vi "ImageAnalysis.vi"(8 "error in (no error)":errorcluster, 10 "config":T5, 11 "data":T1) -> (0 "error out":errorcluster, 3 "data out":T1)   [LabVIEW 2017, in "IrAnalysis.lvlib"]
uses:
  <vilib>/addons/InsightCM/Devices/Shared/Ir/IrAnalysis/IrAnalysis.lvlib
  <vilib>/addons/InsightCM/Devices/Shared/Common/DataFlow/controls/Data.ctl
  <vilib>/addons/InsightCM/Utilities/DataAccessors/controls/wfmSGL_DVR.ctl
  <vilib>/addons/PointValueMap/controls/PointMap.ctl
  <vilib>/addons/InsightCM/Devices/Shared/Common/DataFlow/controls/Type.ctl
  <vilib>/addons/InsightCM/Devices/Shared/Ir/IrAnalysis/controls/config.ctl
  <vilib>/addons/InsightCM/Devices/Shared/Ir/IrAnalysis/controls/roi.ctl
  <vilib>/addons/InsightCM/Devices/Shared/Ir/IrAnalysis/controls/metric.ctl
  <vilib>/addons/InsightCM/MessageBus/Base/controls/MetricDefinitionInstance.ctl
  <vilib>/addons/InsightCM/MessageBus/Base/controls/KeyValuePair.ctl
  <vilib>/addons/PointValueMap/PointValueMap.lvlib
  <vilib>/addons/InsightCM/Devices/Shared/Common/DataFlow/DataFlow.lvlib
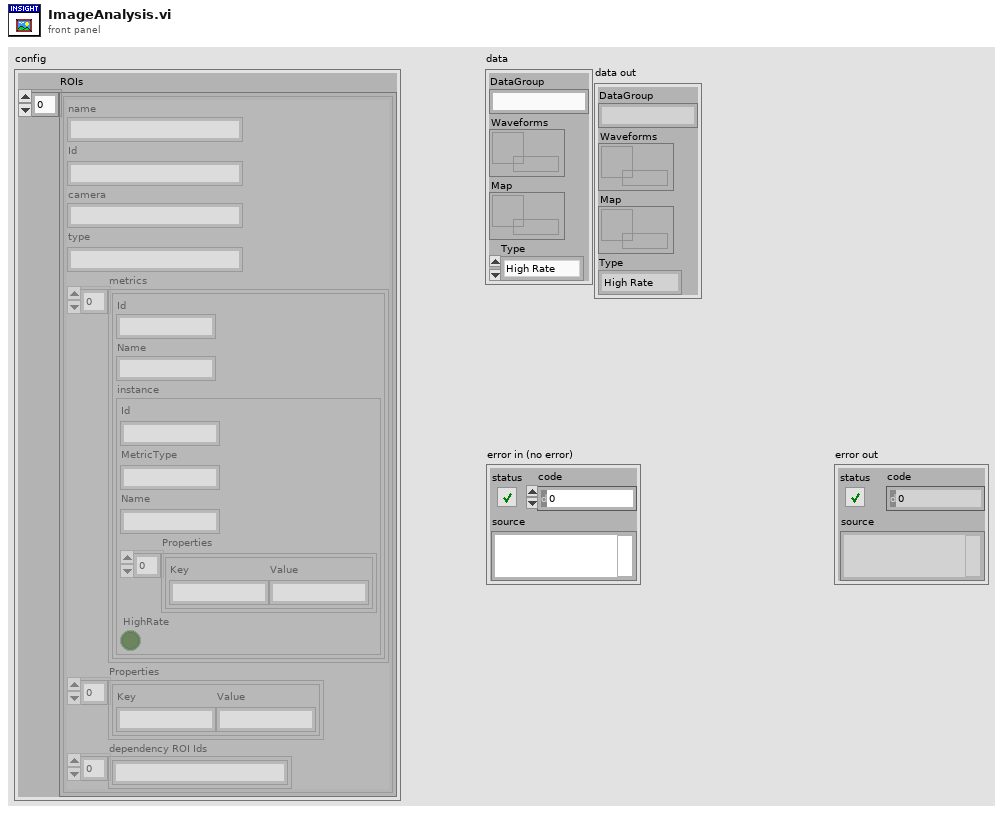
[diagram p1: front panel]
types:
  T1 = typedef "DataFlow.lvlib/Data.ctl" = cluster{"DataGroup":string, "Waveforms":T2, "Map":T3, "Type":T4}
  T2 = typedef "wfmSGL_DVR.ctl" = refnum<data-value>
  T3 = typedef "PointValueMap.lvlib/PointMap.ctl" = refnum<data-value>
  T4 = typedef "DataFlow.lvlib/Type.ctl" = enum16{"High Rate", "Low Rate", "Burst Mode"}
  T5 = typedef "IrAnalysis.lvlib/config.ctl" = cluster{"ROIs":T6[]}
  T6 = typedef "IrAnalysis.lvlib/roi.ctl" = cluster{"name":string, "Id":string, "camera":string, "type":string, "metrics":T7[], "Properties":T9[], "dependency ROI Ids":string[]}
  T7 = typedef "IrAnalysis.lvlib/metric.ctl" = cluster{"Id":string, "Name":string, "instance":T8}
  T8 = typedef "MetricDefinitionInstance.ctl" = cluster{"Id":string, "MetricType":string, "Name":string, "Properties":T9[], "HighRate":bool}
  T9 = typedef "KeyValuePair.ctl" = cluster{"Key":string, "Value":string}
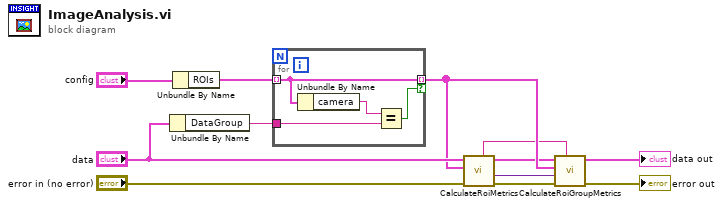
[diagram p0: block diagram]
diagram:
  n1 = Unbundle By Name("data") -> ("DataGroup"=w12:string)
  n2 = Unbundle By Name("config") -> ("ROIs"=w9:T6[])
  n3 = for {
    tunnel: w9 -> [w14] mode=indexing
    tunnel: w12 -> [w15]
    tunnel: [w14] -> w4 mode=indexing if=w13
    n4 = Unbundle By Name(w14) -> ("camera"=w16:string)
    n5 = Equal?(x=w16, y=w15) -> (x = y?=w13:bool)
  }
  n6 = call <vilib>:"CalculateRoiMetrics.vi"("error in (no error)"="error in (no error)", "rois"=w4, "data"="data") -> ("error out"=w8:errorcluster, "roi cache"=w5:variant, "data out"=w3:T1, "image status"=w1:string)  [unwired: 5 in]
  n7 = call <vilib>:"CalculateRoiGroupMetrics.vi"("image status"=w1, "error in (no error)"=w8, "roi cache"=w5, "rois"=w4, "data"=w3) -> ("error out"=→"error out":errorcluster, "data out"=→"data out":T1)  [unwired: 5 in]
